vi "lockinAFMControl.vi"(8 "error in":errorcluster, 10 "NUMERO DE MED.":i32, 11 "milliseconds to wait":u32) -> (0 "error out":errorcluster, 1 "Prom. X":dbl, 2 "X":dbl, 4 "Prom. Y":dbl, 5 "Y":dbl)   [LabVIEW 2018]
uses:
  <vilib>/Instr/_visa.llb/VISA Configure Serial Port (Instr).vi
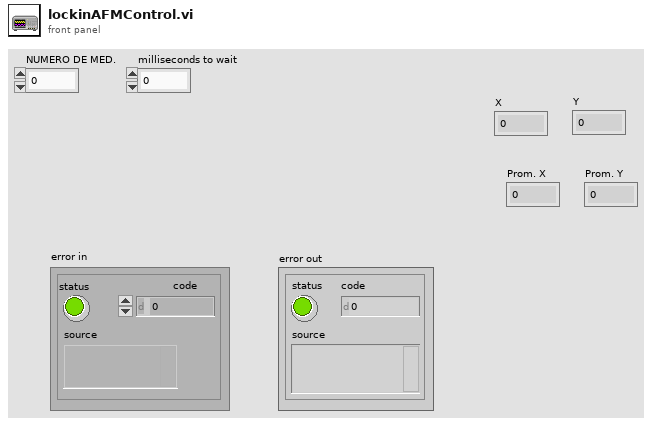
[diagram p1: front panel]
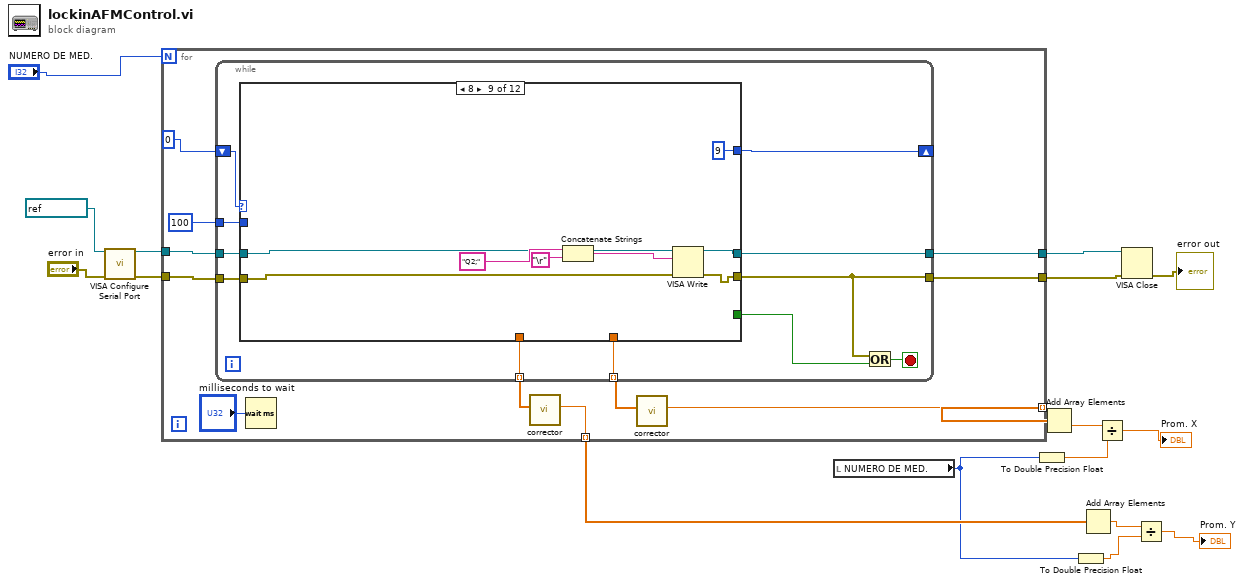
[diagram p0: block diagram]
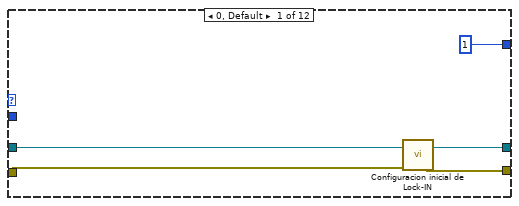
[diagram p2: hidden frame]
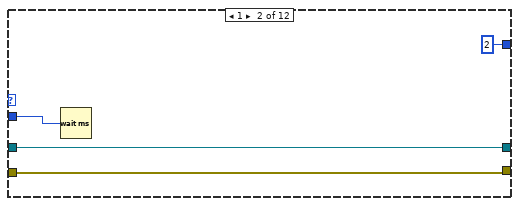
[diagram p3: hidden frame]
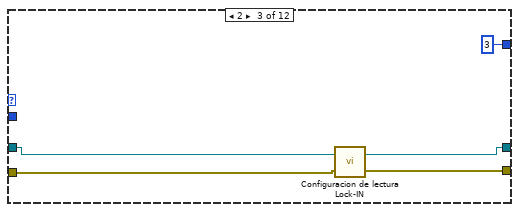
[diagram p4: hidden frame]
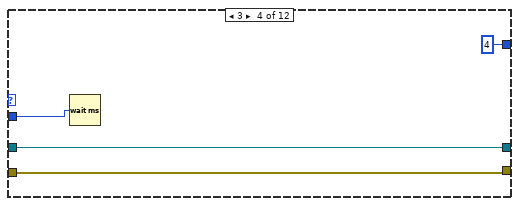
[diagram p5: hidden frame]
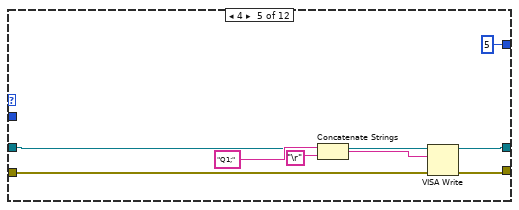
[diagram p6: hidden frame]
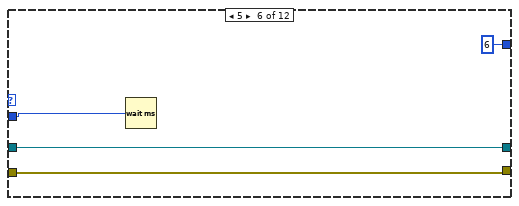
[diagram p7: hidden frame]
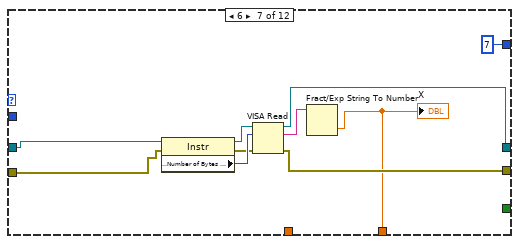
[diagram p8: hidden frame]
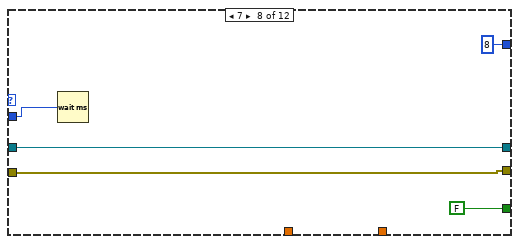
[diagram p9: hidden frame]
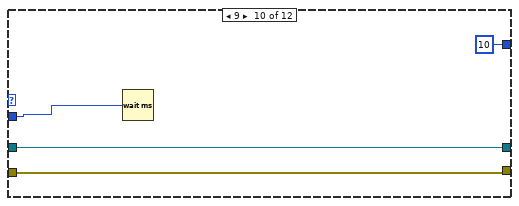
[diagram p10: hidden frame]
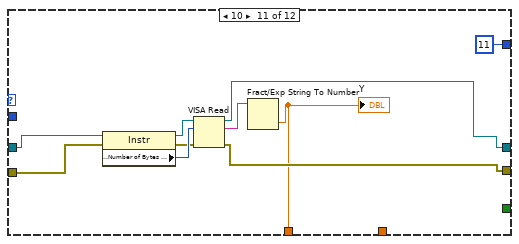
[diagram p11: hidden frame]
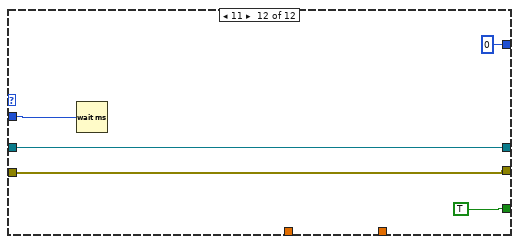
[diagram p12: hidden frame]
diagram:
  n1 = call-poly "VISA Configure Serial Port"("VISA resource name"=refnum<visa-resource-name> "COM4", "error in (no error)"="error in") -> ("VISA resource name out"=w15:refnum<visa-resource-name>, "error out"=w14:errorcluster)  [unwired: 12 in]
  n2 = for {
    N: "NUMERO DE MED." -> [_]
    tunnel: w15 -> [w27]
    tunnel: w14 -> [w26]
    tunnel: [w23] -> w12 mode=indexing
    tunnel: [w21] -> w7
    tunnel: [w20] -> w6
    tunnel: [w18] -> w5 mode=indexing
    n3 = while {
      shift-right: [w35] -> _
      shift-left: 0 -> [w39]
      tunnel: w27 -> [w37]
      tunnel: w26 -> [w36]
      tunnel: 100 -> [w34]
      tunnel: [w33] -> w21
      tunnel: [w32] -> w20
      tunnel: [w30] -> w24 mode=indexing
      tunnel: [w29] -> w19 mode=indexing
      stop <- w38 stop-if-true
      n4 = case shown="8" w39 {
        tunnel: w37 -> [w44 w46 w53 w56 w61 w68 w75 w83 w89 w95 w100 w110]
        tunnel: w36 -> [w43 w45 w52 w55 w60 w67 w74 w82 w88 w94 w99 w109]
        tunnel: [1 2 3 4 5 6 7 8 9 10 11 0] -> w35
        tunnel: w34 -> [_ w48 _ w57 _ w69 _ w84 _ w96 _ w108]
        tunnel: [w41 w46 w51 w56 w62 w68 w73 w83 w86 w95 w102 w110] -> w33
        tunnel: [w40 w45 w50 w55 w59 w67 w72 w82 w87 w94 w101 w109] -> w32
        tunnel: [_ _ _ _ _ _ _ FALSE _ _ _ TRUE] -> w31
        tunnel: [_ _ _ _ _ _ w70 _ _ _ _ _] -> w30
        tunnel: [_ _ _ _ _ _ _ _ _ _ w98 _] -> w29
        frame 0, Default {
          n5 = call "Configuracion inicial de Lock-IN.vi"("error in (no error)"=w43, "VISA resource name"=w44) -> ("error out"=w40:errorcluster, "VISA resource name out"=w41:refnum<visa-resource-name>)
        }
        frame 1 {
          n6 = Wait (ms)(milliseconds to wait=w48) -> ()  [unwired: 1 out]
        }
        frame 2 {
          n7 = call "Configuracion de lectura Lock-IN.vi"("error in (no error)"=w52, "VISA resource name"=w53) -> ("error out"=w50:errorcluster, "VISA resource name out"=w51:refnum<visa-resource-name>)
        }
        frame 3 {
          n8 = Wait (ms)(milliseconds to wait=w57) -> ()  [unwired: 1 out]
        }
        frame 4 {
          n9 = Concatenate Strings("Q1;" ("string"), "\r") -> (w63:string)
          n10 = VISA Write(VISA resource name=w61, write buffer=w63, error in (no error)=w60) -> (VISA resource name out=w62:refnum<visa-resource-name>, error out=w59:errorcluster)  [unwired: 1 out]
        }
        frame 5 {
          n11 = Wait (ms)(milliseconds to wait=w69) -> ()  [unwired: 1 out]
        }
        frame 6 {
          n12 = property class="Instr"(reference=w75, error in=w74) -> (reference out=w79:refnum<visa-resource-name>, error out=w77:errorcluster, "Serial Settings:Number of Bytes at Serial Port"=w78:u32)
          n13 = VISA Read(VISA resource name=w79, byte count=w78, error in (no error)=w77) -> (VISA resource name out=w73:refnum<visa-resource-name>, read buffer=w76:string, error out=w72:errorcluster)  [unwired: 1 out]
          n14 = Fract/Exp String To Number(string=w76) -> (number=w70:dbl)  [unwired: 3 in, 1 out]
          "X" <- w70
        }
        frame 7 {
          n15 = Wait (ms)(milliseconds to wait=w84) -> ()  [unwired: 1 out]
        }
        frame 8 {
          n16 = Concatenate Strings("Q2;" ("string"), "\r") -> (w90:string)
          n17 = VISA Write(VISA resource name=w89, write buffer=w90, error in (no error)=w88) -> (VISA resource name out=w86:refnum<visa-resource-name>, error out=w87:errorcluster)  [unwired: 1 out]
        }
        frame 9 {
          n18 = Wait (ms)(milliseconds to wait=w96) -> ()  [unwired: 1 out]
        }
        frame 10 {
          n19 = property class="Instr"(reference=w100, error in=w99) -> (reference out=w106:refnum<visa-resource-name>, error out=w104:errorcluster, "Serial Settings:Number of Bytes at Serial Port"=w105:u32)
          n20 = VISA Read(VISA resource name=w106, byte count=w105, error in (no error)=w104) -> (VISA resource name out=w102:refnum<visa-resource-name>, read buffer=w103:string, error out=w101:errorcluster)  [unwired: 1 out]
          n21 = Fract/Exp String To Number(string=w103) -> (number=w98:dbl)  [unwired: 3 in, 1 out]
          "Y" <- w98
        }
        frame 11 {
          n22 = Wait (ms)(milliseconds to wait=w108) -> ()  [unwired: 1 out]
        }
      }
      n23 = Or(x=w32, y=w31) -> (x .or. y?=w38:bool)
    }
    n24 = Wait (ms)(milliseconds to wait="milliseconds to wait") -> ()  [unwired: 1 out]
    n25 = call "corrector.vi"("Array"=w19) -> ("valor salida"=w18:dbl)  [unwired: 10 in]
    n26 = call "corrector.vi"("Array"=w24) -> ("valor salida"=w23:dbl)  [unwired: 10 in]
  }
  n27 = local read "NUMERO DE MED."() -> (w2:i32)
  n28 = To Double Precision Float(number=w2) -> (double precision float=w10:dbl)
  n29 = Add Array Elements(numeric array=w12) -> (sum=w11:dbl)
  n30 = To Double Precision Float(number=w2) -> (double precision float=w3:dbl)
  n31 = Add Array Elements(numeric array=w5) -> (sum=w4:dbl)
  n32 = Divide(x=w11, y=w10) -> (x/y=→"Prom. X":dbl)
  n33 = VISA Close(VISA resource name=w7, error in (no error)=w6) -> (error out=→"error out":errorcluster)
  n34 = Divide(x=w4, y=w3) -> (x/y=→"Prom. Y":dbl)
